vi "Open.vi"(8 "error in (no error)":errorcluster, 10 "address":string, 11 "Instrument in":refnum<class "Instrument.lvclass">) -> (0 "error out":errorcluster, 3 "Instrument out":refnum<class "Instrument.lvclass">)   [LabVIEW 2019, in "Instrument.lvlib" / "Instrument.lvclass"]
doc: "Opens a remote connection to an Instrument instance. This can be called on its own or this is called automatically by \"Remote Client.vim\""
uses:
  Instrument.lvclass
  Instrument.lvclass/Instrument.ctl
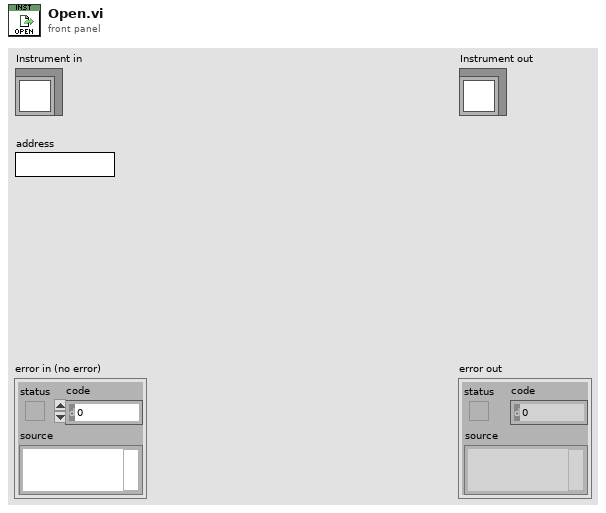
[diagram p1: front panel]
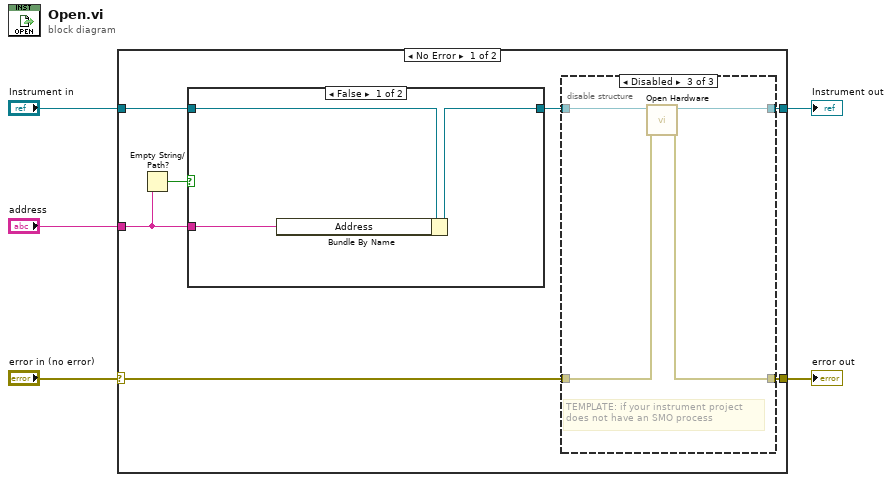
[diagram p0: block diagram]
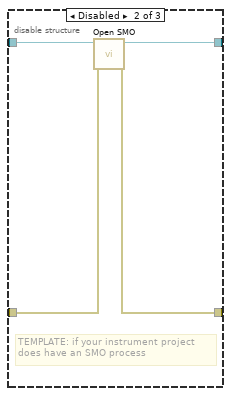
[diagram p4: hidden frame]
diagram:
  n1 = case shown="No Error" "error in (no error)" {
    selector: "error in (no error)" -> [w11 w28]
    tunnel: [w9 w28] -> w4
    tunnel: [w10 w27] -> w2
    tunnel: "Instrument in" -> [w12 w27]
    tunnel: "address" -> [w7 _]
    frame No Error {
      n2 = Empty String/Path?(string/path=w7) -> (empty?=w6:bool)
      n3 = case shown="False" w6 {
        tunnel: w12 -> [w15 w16]
        tunnel: [w14 w16] -> w8
        tunnel: w7 -> [w13 _]
        frame False {
          n4 = Bundle By Name(cluster=w15, "Address"=w13) -> (w14:refnum<class "Instrument.lvclass">)
        }
        frame True {
        }
      }
      n5 = disable-structure shown="Disabled" {
        disable-tunnel: w8 -> [w18 w22 w23]
        disable-tunnel: w11 -> [w17 w20 w25]
        disable-tunnel: [w18 w21 w26] -> w10
        disable-tunnel: [w17 w19 w24] -> w9
        frame Enabled {
        }
        frame Disabled {
          # "TEMPLATE: if your instrument project\ndoes have an SMO process"
          n6 = call "Open SMO.vi"("error in (no error)"=w20, "Instrument in"=w22) -> ("error out"=w19:errorcluster, "Instrument out"=w21:refnum<class "Instrument.lvclass">)  [unwired: 8 in]
        }
        frame Disabled {
          # "TEMPLATE: if your instrument project\ndoes not have an SMO process"
          n7 = call-dynamic "Open Hardware.vi"("error in (no error)"=w25, "Instrument in"=w23) -> ("error out"=w24:errorcluster, "Instrument out"=w26:refnum<class "Instrument.lvclass">)  [unwired: 8 in]
        }
      }
    }
    frame Error {
    }
  }
  "error out" <- w4
  "Instrument out" <- w2
